vi "WS1050_AD7747_Control_Cap_bank_Measure Debug.vi"(0 "Select Com Port":refnum<visa-resource-name>="COM1", 1 "Click down to quit":bool=TRUE, 2 "Push Button to Initialize AD7747":bool, 3 "Push Button to Calibrate":bool, 7 "Push Button to write Offset":bool, 11 "errorin":errorcluster, 12 "Push Button to Measue Cap":bool=TRUE, 13 "CApDac_values":string[](array[string])=["900b89", "900b89", "900b89"]) -> (4 "C2L(pF)":dbl, 8 "C1L(pF)":dbl, 10 "C3L(pF)":dbl, 14 "Com Port Out":refnum<visa-resource-name>="COM1", 15 "error out":errorcluster)   [LabVIEW 2012]
panel:
  out "C3L_Mesa(pF)":dbl
  out "C2L_Mesa(pF)":dbl
  out "C1L_Mesa(pF)":dbl
  # "AD7747 Control Ver1.0"
  # "Interface PIC I2C Control"
  # "Bank Cap Measurements"
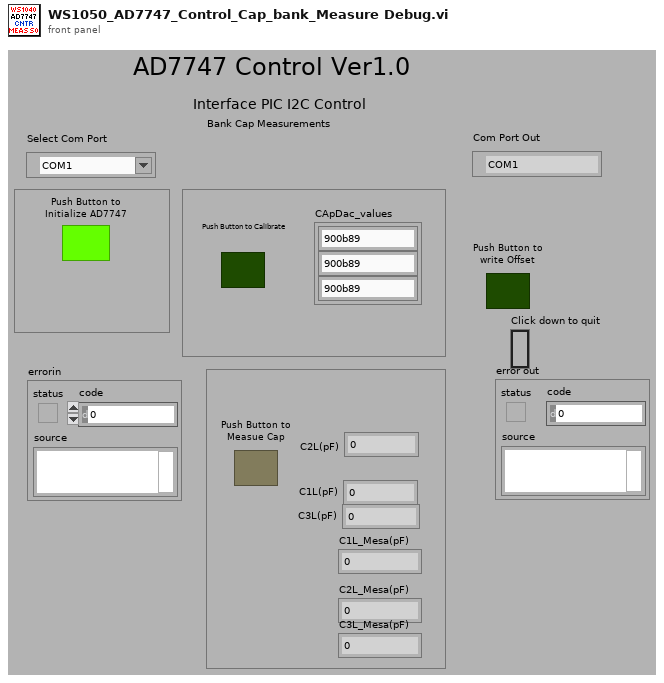
[diagram p1: front panel]
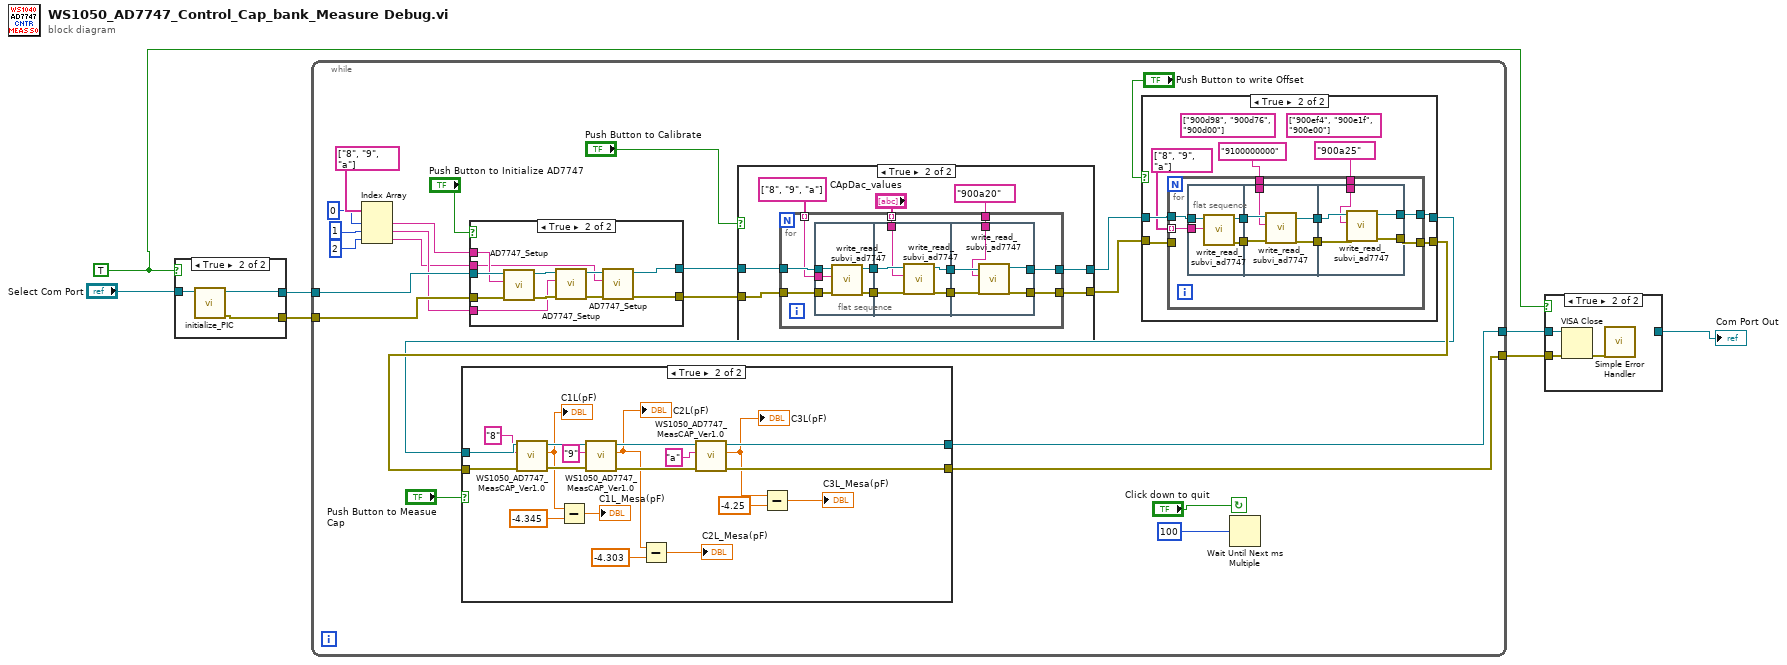
[diagram p0: block diagram]
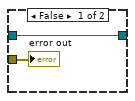
[diagram p2: hidden frame]
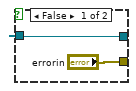
[diagram p3: hidden frame]
diagram:
  w2 = TRUE
  n1 = case shown="True" w2 {
    tunnel: ["errorin" w12] -> w7
    tunnel: [w8 w11] -> w6
    tunnel: "Select Com Port" -> [w8 w10]
    frame False {
    }
    frame True {
      n2 = call "initialize_PIC.vi"("Select Com Port"=w10) -> ("error out"=w12:errorcluster, "VISA resource name out"=w11:refnum<visa-resource-name>)  [unwired: 9 in]
    }
  }
  n3 = while {
    tunnel: w7 -> [w30]
    tunnel: w6 -> [w28]
    tunnel: [w17] -> w5
    tunnel: [w35] -> w4
    stop <- "Click down to quit" continue-if-true
    n4 = Index Array(array=string[] ["8", "9", "a"], index #1=0 ("index"), index #2=1 ("index"), index #3=2 ("index")) -> (element #1=w31:string, element #2=w24:string, element #3=w23:string)
    n5 = case shown="True" "Push Button to Initialize AD7747" {
      tunnel: w30 -> [w104 w115]
      tunnel: [w104 w105] -> w18
      tunnel: w28 -> [w103 w114]
      tunnel: w31 -> [_ w109]
      tunnel: w24 -> [_ w108]
      tunnel: w23 -> [_ w107]
      tunnel: [w103 w106] -> w15
      frame False {
      }
      frame True {
        n6 = call "AD7747_Setup.vi"("error in"=w115, "AD7747_Number"=w109, "Control"=w114) -> ("error out"=w113:errorcluster, "Control out"=w112:refnum<visa-resource-name>)  [unwired: 6 in, 1 out]
        n7 = call "AD7747_Setup.vi"("error in"=w113, "AD7747_Number"=w108, "Control"=w112) -> ("error out"=w111:errorcluster, "Control out"=w110:refnum<visa-resource-name>)  [unwired: 6 in, 1 out]
        n8 = call "AD7747_Setup.vi"("error in"=w111, "AD7747_Number"=w107, "Control"=w110) -> ("error out"=w105:errorcluster, "Control out"=w106:refnum<visa-resource-name>)  [unwired: 6 in, 1 out]
      }
    }
    n9 = case shown="True" "Push Button to Calibrate" {
      tunnel: [w69 w77] -> w29
      tunnel: w18 -> [w69 w74]
      tunnel: w15 -> [w70 w73]
      tunnel: [w70 w72] -> w14
      frame False {
      }
      frame True {
        n10 = for {
          tunnel: [w83] -> w77
          tunnel: w73 -> [w87]
          tunnel: w74 -> [w88]
          tunnel: string[] ["8", "9", "a"] -> [w86] mode=indexing
          tunnel: "CApDac_values" -> [w82] mode=indexing
          tunnel: [w81] -> w72
          tunnel: "900a20" ("Data_In 2") -> [w78]
          n11 = flat-sequence {
            tunnel: w88 -> [w93]
            tunnel: w87 -> [w91]
            tunnel: w86 -> [w89]
            tunnel: [w92] -> w85
            tunnel: [w90] -> w84
            tunnel: w85 -> [w97]
            tunnel: w84 -> [w98]
            tunnel: w82 -> [w95]
            tunnel: [w96] -> w80
            tunnel: [w94] -> w79
            tunnel: [w100] -> w81
            tunnel: [w102] -> w83
            tunnel: w80 -> [w102]
            tunnel: w79 -> [w101]
            tunnel: w78 -> [w99]
            frame #0 {
              n12 = call "write_read_subvi_ad7747.vi"("error in (no error)"=w93, "command"=w89, "Control"=w91) -> ("error out"=w92:errorcluster, "Control out"=w90:refnum<visa-resource-name>)  [unwired: 6 in, 1 out]
            }
            frame #1 {
              n13 = call "write_read_subvi_ad7747.vi"("error in (no error)"=w97, "command"=w95, "Control"=w98) -> ("error out"=w96:errorcluster, "Control out"=w94:refnum<visa-resource-name>)  [unwired: 6 in, 1 out]
            }
            frame #2 {
              n14 = call "write_read_subvi_ad7747.vi"("command"=w99, "Control"=w101) -> ("Control out"=w100:refnum<visa-resource-name>)  [unwired: 7 in, 2 out]
            }
          }
        }
      }
    }
    n15 = case shown="True" "Push Button to write Offset" {
      tunnel: w14 -> [w36 w43]
      tunnel: w29 -> [w37 w44]
      tunnel: [w37 w41] -> w16
      tunnel: [w36 w40] -> w13
      frame False {
      }
      frame True {
        (unwired) string[] ["900ef4", "900e1f", "900e00"]
        (unwired) string[] ["900d98", "900d76", "900d00"]
        n16 = for {
          tunnel: w44 -> [_]
          tunnel: [w48] -> w41
          tunnel: w43 -> [w54]
          tunnel: string[] ["8", "9", "a"] -> [w53] mode=indexing
          tunnel: "9100000000" ("Data_In 2") -> [w47]
          tunnel: "900a25" ("Data_In 2") -> [w46]
          tunnel: [w45] -> w40
          n17 = flat-sequence {
            tunnel: w54 -> [w56]
            tunnel: w53 -> [w55]
            tunnel: [w58] -> w52
            tunnel: [w57] -> w51
            tunnel: w52 -> [w61]
            tunnel: w51 -> [w63]
            tunnel: [w60] -> w50
            tunnel: [w62] -> w49
            tunnel: w47 -> [w59]
            tunnel: w50 -> [w67]
            tunnel: w49 -> [w68]
            tunnel: [w66] -> w48
            tunnel: w46 -> [w65]
            tunnel: [w64] -> w45
            frame #0 {
              n18 = call "write_read_subvi_ad7747.vi"("command"=w55, "Control"=w56) -> ("error out"=w58:errorcluster, "Control out"=w57:refnum<visa-resource-name>)  [unwired: 7 in, 1 out]
            }
            frame #1 {
              n19 = call "write_read_subvi_ad7747.vi"("error in (no error)"=w61, "command"=w59, "Control"=w63) -> ("error out"=w60:errorcluster, "Control out"=w62:refnum<visa-resource-name>)  [unwired: 6 in, 1 out]
            }
            frame #2 {
              n20 = call "write_read_subvi_ad7747.vi"("error in (no error)"=w67, "command"=w65, "Control"=w68) -> ("error out"=w66:errorcluster, "Control out"=w64:refnum<visa-resource-name>)  [unwired: 6 in, 1 out]
            }
          }
        }
      }
    }
    n21 = case shown="True" "Push Button to Measue Cap" {
      tunnel: w16 -> [w117 w137]
      tunnel: w13 -> [w116 w136]
      tunnel: [w117 w128] -> w17
      tunnel: [w116 w127] -> w35
      frame False {
      }
      frame True {
        n22 = call "WS1050_AD7747_MeasCAP_Ver1.0.vi"("error in (no error)"=w137, "AD7747_Number"="8", "Control"=w136) -> ("error"=w133:errorcluster, "CAP (pF)"=w125:dbl, "Control out"=w132:refnum<visa-resource-name>)  [unwired: 5 in, 1 out]
        "C1L(pF)" <- w125
        n23 = Subtract(x=w125, y=-4.345) -> (x-y=→"C1L_Mesa(pF)":dbl)
        n24 = call "WS1050_AD7747_MeasCAP_Ver1.0.vi"("error in (no error)"=w133, "AD7747_Number"="9", "Control"=w132) -> ("error"=w130:errorcluster, "CAP (pF)"=w122:dbl, "Control out"=w129:refnum<visa-resource-name>)  [unwired: 5 in, 1 out]
        "C2L(pF)" <- w122
        n25 = Subtract(x=w122, y=-4.303) -> (x-y=→"C2L_Mesa(pF)":dbl)
        n26 = call "WS1050_AD7747_MeasCAP_Ver1.0.vi"("error in (no error)"=w130, "AD7747_Number"="a", "Control"=w129) -> ("error"=w128:errorcluster, "CAP (pF)"=w119:dbl, "Control out"=w127:refnum<visa-resource-name>)  [unwired: 5 in, 1 out]
        "C3L(pF)" <- w119
        n27 = Subtract(x=w119, y=-4.25) -> (x-y=→"C3L_Mesa(pF)":dbl)
      }
    }
    n28 = Wait Until Next ms Multiple(millisecond multiple=u32 100) -> ()  [unwired: 1 out]
  }
  n29 = case shown="True" w2 {
    tunnel: w5 -> [w139 w141]
    tunnel: w4 -> [w138 w140]
    tunnel: [w138 _] -> w1
    frame False {
      "error out" <- w139
    }
    frame True {
      n30 = VISA Close(VISA resource name=w140, error in (no error)=w141) -> (error out=w142:errorcluster)
      n31 = call <vilib>:"Simple Error Handler.vi"("error in (no error)"=w142) -> ()  [unwired: 1 in, 8 out]
    }
  }
  "Com Port Out" <- w1
